vi "dcy06.vi"() -> ()   [LabVIEW 2015]
uses:
  SECoP.lvlib
  <vilib>/regexp/Match Regular Expression.xnode
  Public/SECoP-data/SECoP-data.ctl
  Public/SECoP-action.ctl
  parametertype.ctl
panel:
  out "log":string
  in  "DLL path":path=path "C:/Users/user/Desktop/x86_64"
  in  "stop":bool
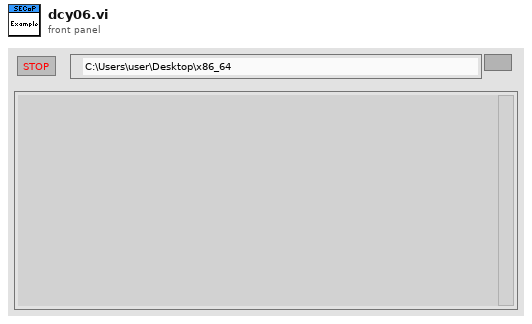
[diagram p1: front panel]
types:
  T1 = typedef "parametertype.ctl" = enum8{"readonly", "readwrite", "command"}
  T2 = typedef "SECoP.lvlib/SECoP-data.ctl" = cluster{"ptr32":u32, "ptr64":u64}
  T3 = cluster{"name":string, "type":T1, "datatype":string, "description":string, "SECoP_dataPtr":T2}[]
  T4 = typedef "SECoP.lvlib/SECoP-libraries.ctl" = cluster{"serverDLL":path, "variantDLL":path, "cleanup_mode":bool}
  T5 = cluster{"name":string, "type":T1, "datatype":string, "description":string, "SECoP_dataPtr":T2}
  T6 = typedef "SECoP.lvlib/SECoP-action.ctl" = enum32{"any action", "read", "change", "do cmd"}
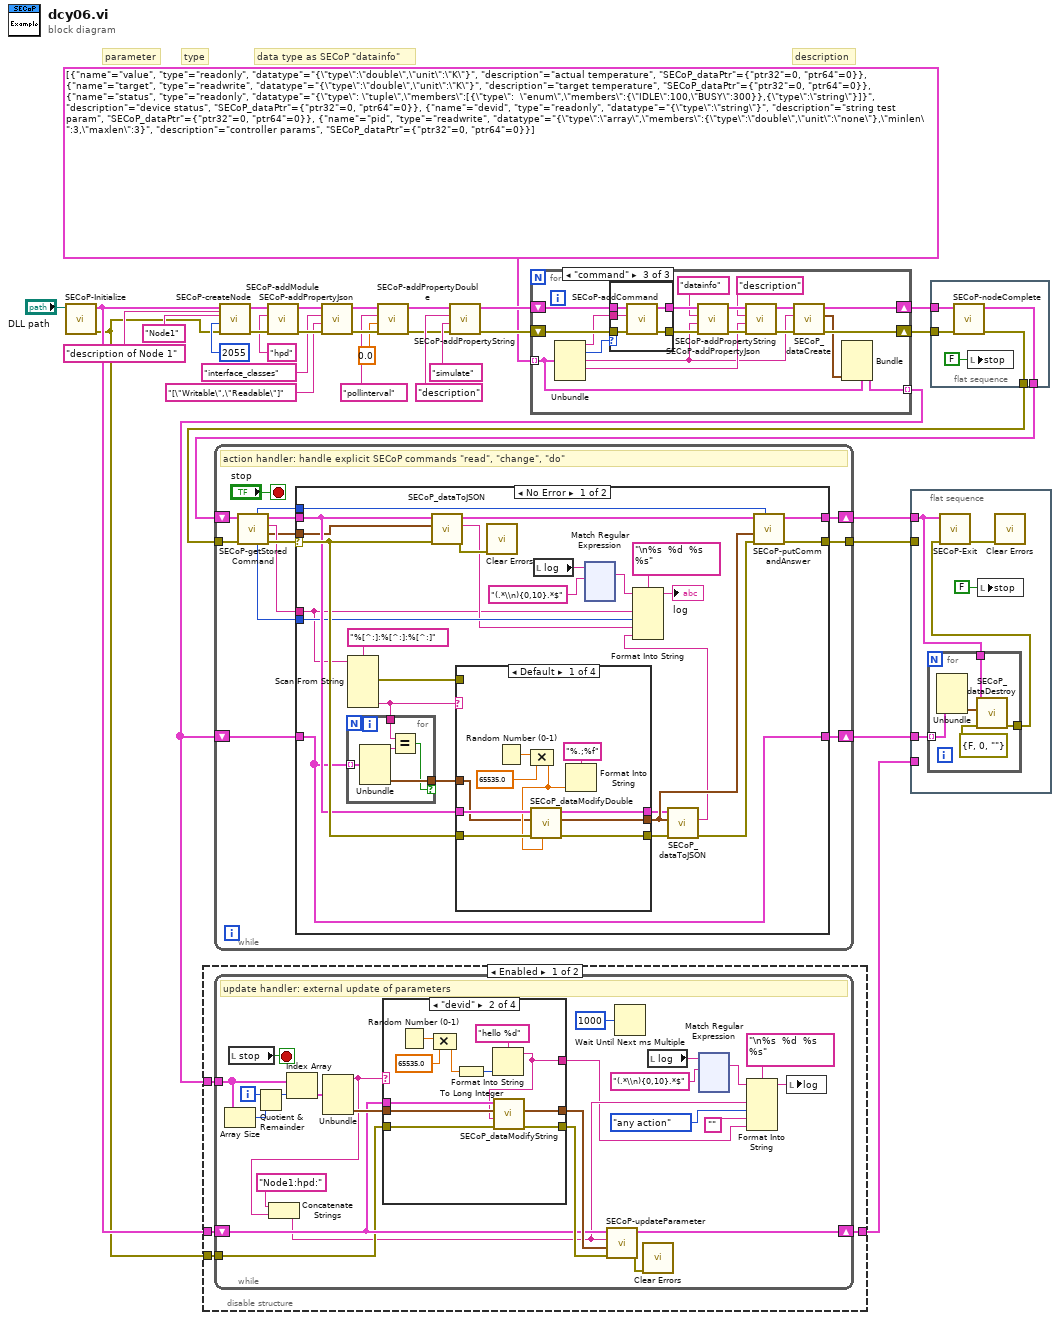
[diagram p0: block diagram]
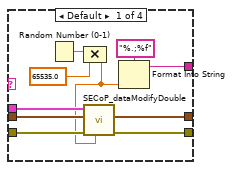
[diagram p2: hidden frame]
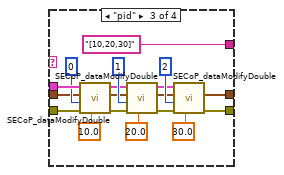
[diagram p3: hidden frame]
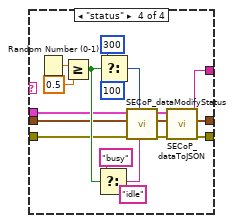
[diagram p4: hidden frame]
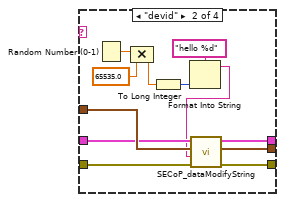
[diagram p6: hidden frame]
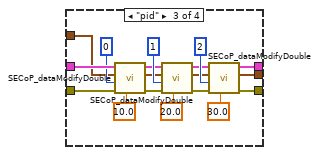
[diagram p7: hidden frame]
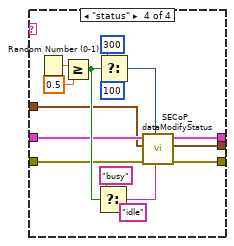
[diagram p8: hidden frame]
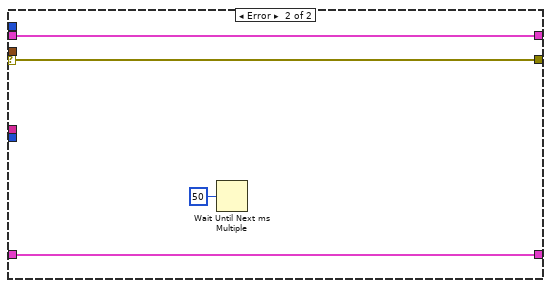
[diagram p9: hidden frame]
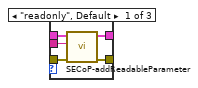
[diagram p10: hidden frame]
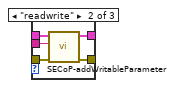
[diagram p11: hidden frame]
diagram:
  # "description"
  # "data type as SECoP \"datainfo\""
  # "type"
  # "parameter"
  n1 = call "SECoP-Initialize.vi"("DLL path (in)"="DLL path") -> ("error out"=w3:errorcluster, "DLL path (out)"=w4:T4)  [unwired: 9 in]
  n2 = call "SECoP-createNode.vi"("description"="description of Node 1", "error in (no error)"=w3, "TCP port"=u16 2055, "node id"="Node1" ("id"), "DLL path (in)"=w4) -> ("error out"=w28:errorcluster, "DLL path (out)"=w32:T4)  [unwired: 5 in]
  n3 = call "SECoP-addModule.vi"("error in (no error)"=w28, "module name"="hpd" ("name"), "DLL path (in)"=w32) -> ("error out"=w25:errorcluster, "DLL path (out)"=w26:T4)  [unwired: 7 in]
  n4 = call "SECoP-addPropertyJson.vi"("error in (no error)"=w25, "property value"="[\"Writable\",\"Readable\"]" ("name"), "property name"="interface_classes" ("name"), "DLL path (in)"=w26) -> ("error out"=w14:errorcluster, "DLL path (out)"=w16:T4)  [unwired: 6 in]
  n5 = call "SECoP-addPropertyDouble.vi"("error in (no error)"=w14, "property value"=0.0, "property name"="pollinterval", "DLL path (in)"=w16) -> ("error out"=w13:errorcluster, "DLL path (out)"=w15:T4)  [unwired: 6 in]
  n6 = call "SECoP-addPropertyString.vi"("error in (no error)"=w13, "property value"="simulate" ("name"), "property name"="description" ("name"), "DLL path (in)"=w15) -> ("error out"=w19:errorcluster, "DLL path (out)"=w20:T4)  [unwired: 6 in]
  n7 = for {
    tunnel: T3 [{"name"="value", "type"=enum."readonly", "datatype"="{\"type\":\"double\",\"unit\":\"K\"}", "description"="actual temperature", "SECoP_dataPtr"={"ptr32"=0, "ptr64"=0}}, {"name"="target", "type"=enum."readwrite", "datatype"="{\"type\":\"double\",\"unit\":\"K\"}", "description"="target temperature", "SECoP_dataPtr"={"ptr32"=0, "ptr64"=0}}, {"name"="status", "type"=enum."readonly", "datatype"="{\"type\": \"tuple\",\"members\":[{\"type\":  \"enum\",\"members\":{\"IDLE\":100,\"BUSY\":300}},{\"type\":\"string\"}]}", "description"="device status", "SECoP_dataPtr"={"ptr32"=0, "ptr64"=0}}, {"name"="devid", "type"=enum."readonly", "datatype"="{\"type\":\"string\"}", "description"="string test param", "SECoP_dataPtr"={"ptr32"=0, "ptr64"=0}}, {"name"="pid", "type"=enum."readwrite", "datatype"="{\"type\":\"array\",\"members\":{\"type\":\"double\",\"unit\":\"none\"},\"minlen\":3,\"maxlen\":3}", "description"="controller params", "SECoP_dataPtr"={"ptr32"=0, "ptr64"=0}}] -> [w36] mode=indexing
    shift-right: [w39] -> w8
    shift-left: w20 -> [w49]
    shift-right: [w38] -> w7
    shift-left: w19 -> [w48]
    tunnel: [w34] -> w1 mode=indexing
    n8 = Unbundle(w36) -> ("name"=w37:string, "type"=w50:T1, "datatype"=w40:string, "description"=w43:string)  [unwired: 1 out]
    n9 = case shown="\"command\"" w50 {
      tunnel: w37 -> [w55 w62 w67]
      tunnel: w49 -> [w57 w61 w66]
      tunnel: [w56 w60 w65] -> w47
      tunnel: [w53 w58 w63] -> w46
      tunnel: w48 -> [w54 w59 w64]
      frame "readonly", Default {
        n10 = call "SECoP-addReadableParameter.vi"("error in (no error)"=w54, "parameter name"=w55, "DLL path (in)"=w57) -> ("error out"=w53:errorcluster, "DLL path (out)"=w56:T4)  [unwired: 7 in]
      }
      frame "readwrite" {
        n11 = call "SECoP-addWritableParameter.vi"("error in (no error)"=w59, "parameter name"=w62, "DLL path (in)"=w61) -> ("error out"=w58:errorcluster, "DLL path (out)"=w60:T4)  [unwired: 7 in]
      }
      frame "command" {
        n12 = call "SECoP-addCommand.vi"("error in (no error)"=w64, "command name"=w67, "DLL path (in)"=w66) -> ("error out"=w63:errorcluster, "DLL path (out)"=w65:T4)  [unwired: 7 in]
      }
    }
    n13 = call "SECoP-addPropertyJson.vi"("error in (no error)"=w46, "property value"=w40, "property name"="datainfo" ("name"), "DLL path (in)"=w47) -> ("error out"=w51:errorcluster, "DLL path (out)"=w52:T4)  [unwired: 6 in]
    n14 = call "SECoP-addPropertyString.vi"("error in (no error)"=w51, "property value"=w43, "property name"="description" ("name"), "DLL path (in)"=w52) -> ("error out"=w42:errorcluster, "DLL path (out)"=w41:T4)  [unwired: 6 in]
    n15 = call "SECoP_dataCreate.vi"("error in (no error)"=w42, "Description"=w40, "DLL path (in)"=w41) -> ("error out"=w38:errorcluster, "SECoP_dataPtr (out)"=w35:T2, "DLL path (out)"=w39:T4)  [unwired: 6 in]
    n16 = Bundle(cluster=w36, "SECoP_dataPtr"=w35) -> (w34:T5)  [unwired: 4 in]
  }
  n17 = disable-structure shown="Enabled" {
    disable-tunnel: [w71 w261] -> w5
    disable-tunnel: w4 -> [w70 w261]
    disable-tunnel: w3 -> [w69 _]
    disable-tunnel: w1 -> [w68 _]
    frame Enabled {
      n18 = while {
        tunnel: w69 -> [w91]
        shift-right: [w90] -> w71
        shift-left: w70 -> [w92]
        tunnel: w68 -> [w81]
        i -> [w83]
        stop <- w93 stop-if-true
        # "update handler: external update of parameters"
        n19 = Array Size(array=w81) -> (size(s)=w84:i32)
        n20 = local read "stop"() -> (w93:bool)
        n21 = Quotient & Remainder(x=w83, y=w84) -> (x-y*floor(x/y)=w85:i32)  [unwired: 1 out]
        n22 = Index Array(array=w81, index=w85) -> (element=w82:T5)
        n23 = Unbundle(w82) -> ("name"=w88:string, "SECoP_dataPtr"=w94:T2)  [unwired: 3 out]
        n24 = Concatenate Strings("Node1:hpd:" ("string"), w88) -> (w76:string)
        n25 = case shown="\"devid\"" w88 {
          tunnel: [w215 w221 "[10,20,30]" w247] -> w74
          tunnel: w92 -> [w214 w225 w244 w252]
          tunnel: [w219 w222 w230 w250] -> w95
          tunnel: w91 -> [w213 w224 w242 w251]
          tunnel: [w212 w223 w231 w253] -> w96
          tunnel: w94 -> [w219 w222 w230 w250]
          frame Default {
            n26 = Random Number (0-1)() -> (number: 0 to 1=w217:dbl)
            n27 = Compound Arithmetic op=MULTIPLY(w217, 65535.0 ("value")) -> (w211:dbl)
            n28 = call "SECoP_dataModifyDouble.vi"("Value"=w211, "error in (no error)"=w213, "SECoP_data"=w219, "DLL path (in)"=w214) -> ("error out"=w212:errorcluster)  [unwired: 6 in, 1 out]
            n29 = Format Into String(format string="%.;%f", w211) -> (resulting string=w215:string)  [unwired: 2 in, 1 out]
          }
          frame "devid" {
            n30 = Random Number (0-1)() -> (number: 0 to 1=w226:dbl)
            n31 = Compound Arithmetic op=MULTIPLY(w226, 65535.0 ("value")) -> (w228:dbl)
            n32 = To Long Integer(number=w228) -> (32bit integer=w229:i32)
            n33 = Format Into String(format string="hello %d", w229) -> (resulting string=w221:string)  [unwired: 2 in, 1 out]
            n34 = call "SECoP_dataModifyString.vi"("error in (no error)"=w224, "Value"=w221, "SECoP_dataPtr"=w222, "DLL path (in)"=w225) -> ("error out"=w223:errorcluster)  [unwired: 6 in, 1 out]
          }
          frame "pid" {
            n35 = call "SECoP_dataModifyDouble.vi"("Value"=10.0, "error in (no error)"=w242, "Index"=u32 0, "SECoP_data"=w230, "DLL path (in)"=w244) -> ("error out"=w233:errorcluster, "DLL path (out)"=w235:T4)  [unwired: 5 in]
            n36 = call "SECoP_dataModifyDouble.vi"("Value"=20.0, "error in (no error)"=w233, "Index"=u32 1, "SECoP_data"=w230, "DLL path (in)"=w235) -> ("error out"=w232:errorcluster, "DLL path (out)"=w234:T4)  [unwired: 5 in]
            n37 = call "SECoP_dataModifyDouble.vi"("Value"=30.0, "error in (no error)"=w232, "Index"=u32 2, "SECoP_data"=w230, "DLL path (in)"=w234) -> ("error out"=w231:errorcluster)  [unwired: 5 in, 1 out]
          }
          frame "status" {
            n38 = Random Number (0-1)() -> (number: 0 to 1=w260:dbl)
            n39 = Greater Or Equal?(x=w260, y=0.5) -> (x >= y?=w256:bool)
            n40 = Select(t="busy", s=w256, f="idle") -> (s? t:f=w246:string)
            n41 = Select(t=i64 300 ("Value"), s=w256, f=i64 100 ("Value")) -> (s? t:f=w245:i64)
            n42 = call "SECoP_dataModifyStatus.vi"("status text"=w246, "status code"=w245, "error in (no error)"=w251, "SECoP_dataPtr (in)"=w250, "DLL path (in)"=w252) -> ("error out"=w248:errorcluster, "DLL path (out)"=w249:T4)  [unwired: 4 in, 1 out]
            n43 = call "SECoP_dataToJSON.vi"("error in (no error)"=w248, "SECoP_dataPtr"=w250, "DLL path (in)"=w249) -> ("error out"=w253:errorcluster, "JSONBuffer"=w247:string)  [unwired: 6 in, 1 out]
          }
        }
        n44 = call "SECoP-updateParameter.vi"("error in (no error)"=w96, "value (SECoP_data)"=w95, "parameter name"=w76, "DLL path (in)"=w92) -> ("error out"=w86:errorcluster, "DLL path (out)"=w90:T4)  [unwired: 6 in]
        n45 = Wait Until Next ms Multiple(millisecond multiple=u32 1000) -> ()  [unwired: 1 out]
        n46 = call <vilib>:"Clear Errors.vi"("error in (no error)"=w86) -> ()  [unwired: 5 in, 2 out]
        n47 = local read "log"() -> (w80:string)
        n48 = xnode "Match Regular Expression"("input string"=w80, "regular expression"="(.*\\n){0,10}.*$") -> ("whole match"=w79:string)  [unwired: 4 in, 4 out]
        n49 = Format Into String(format string="\n%s  %d  %s  %s", initial string=w79, w76, SECoP-action."any action" ("input 2"), "", w74) -> (resulting string=w72:string)  [unwired: 1 in, 1 out]
        n50 = local write "log"(w72) -> ()
      }
    }
    frame Disabled {
    }
  }
  n51 = while {
    shift-right: [w274] -> w22
    shift-left: w9 -> [w272]
    tunnel: w10 -> [w271]
    tunnel: [w264] -> w21
    shift-right: [w262] -> w6
    shift-left: w1 -> [w263]
    stop <- "stop" stop-if-true
    # "action handler: handle explicit SECoP commands \"read\", \"change\", \"do\""
    n52 = call "SECoP-getStoredCommand.vi"("error in (no error)"=w271, "DLL path (in)"=w272) -> ("error out"=w269:errorcluster, "SECoP_data"=w265:T2, "command/parameter path"=w266:string, "DLL path (out)"=w270:T4, "action"=w267:T6, "command id"=w268:u64)  [unwired: 4 in]
    n53 = case shown="No Error" w269 {
      selector: w269 -> [w299 w471]
      tunnel: w270 -> [w298 w472]
      tunnel: [w295 w472] -> w274
      tunnel: w268 -> [w294 _]
      tunnel: w266 -> [w283 _]
      tunnel: w265 -> [w280 _]
      tunnel: w267 -> [w293 _]
      tunnel: [w296 w471] -> w264
      tunnel: w263 -> [w279 w470]
      tunnel: [w279 w470] -> w262
      frame No Error {
        n54 = Scan From String(format string="%[^:]:%[^:]:%[^:]", input string=w283) -> (error out=w287:errorcluster, output 3=w282:string)  [unwired: 7 in, 2 out]
        n55 = for {
          tunnel: w279 -> [w301] mode=indexing
          tunnel: w282 -> [w304]
          tunnel: [w303] -> w281 if=w302
          n56 = Unbundle(w301) -> ("name"=w305:string, "SECoP_dataPtr"=w303:T2)  [unwired: 3 out]
          n57 = Equal?(x=w304, y=w305) -> (x = y?=w302:bool)
        }
        n58 = call "SECoP_dataToJSON.vi"("error in (no error)"=w299, "SECoP_dataPtr"=w280, "DLL path (in)"=w298) -> ("error out"=w297:errorcluster, "JSONBuffer"=w284:string, "DLL path (out)"=w285:T4)  [unwired: 6 in]
        n59 = case shown="Default" w282 {
          tunnel: w287 -> [_ _ _ _]
          tunnel: w298 -> [w311 w319 w340 w347]
          tunnel: [w307 w325 w327 w345] -> w300
          tunnel: w299 -> [w310 w318 w339 w346]
          tunnel: [w309 w316 w328 w342] -> w276
          tunnel: w281 -> [w307 w325 w327 w345]
          tunnel: [w306 w315 w326 w341] -> w277
          frame Default {
            n60 = Random Number (0-1)() -> (number: 0 to 1=w313:dbl)
            n61 = Compound Arithmetic op=MULTIPLY(w313, 65535.0 ("value")) -> (w308:dbl)
            n62 = call "SECoP_dataModifyDouble.vi"("Value"=w308, "error in (no error)"=w310, "SECoP_data"=w307, "DLL path (in)"=w311) -> ("error out"=w309:errorcluster, "DLL path (out)"=w306:T4)  [unwired: 6 in]
            n63 = Format Into String(format string="%.;%f", w308) -> ()  [unwired: 2 in, 2 out]
          }
          frame "devid" {
            n64 = Random Number (0-1)() -> (number: 0 to 1=w321:dbl)
            n65 = Compound Arithmetic op=MULTIPLY(w321, 65535.0 ("value")) -> (w323:dbl)
            n66 = To Long Integer(number=w323) -> (32bit integer=w324:i32)
            n67 = Format Into String(format string="hello %d", w324) -> (resulting string=w317:string)  [unwired: 2 in, 1 out]
            n68 = call "SECoP_dataModifyString.vi"("error in (no error)"=w318, "Value"=w317, "SECoP_dataPtr"=w325, "DLL path (in)"=w319) -> ("error out"=w316:errorcluster, "DLL path (out)"=w315:T4)  [unwired: 6 in]
          }
          frame "pid" {
            n69 = call "SECoP_dataModifyDouble.vi"("Value"=10.0, "error in (no error)"=w339, "Index"=u32 0, "SECoP_data"=w327, "DLL path (in)"=w340) -> ("error out"=w330:errorcluster, "DLL path (out)"=w332:T4)  [unwired: 5 in]
            n70 = call "SECoP_dataModifyDouble.vi"("Value"=20.0, "error in (no error)"=w330, "Index"=u32 1, "SECoP_data"=w327, "DLL path (in)"=w332) -> ("error out"=w329:errorcluster, "DLL path (out)"=w331:T4)  [unwired: 5 in]
            n71 = call "SECoP_dataModifyDouble.vi"("Value"=30.0, "error in (no error)"=w329, "Index"=u32 2, "SECoP_data"=w327, "DLL path (in)"=w331) -> ("error out"=w328:errorcluster, "DLL path (out)"=w326:T4)  [unwired: 5 in]
          }
          frame "status" {
            n72 = Random Number (0-1)() -> (number: 0 to 1=w354:dbl)
            n73 = Greater Or Equal?(x=w354, y=0.5) -> (x >= y?=w350:bool)
            n74 = Select(t="busy", s=w350, f="idle") -> (s? t:f=w344:string)
            n75 = Select(t=i64 300 ("Value"), s=w350, f=i64 100 ("Value")) -> (s? t:f=w343:i64)
            n76 = call "SECoP_dataModifyStatus.vi"("status text"=w344, "status code"=w343, "error in (no error)"=w346, "SECoP_dataPtr (in)"=w345, "DLL path (in)"=w347) -> ("error out"=w342:errorcluster, "DLL path (out)"=w341:T4)  [unwired: 4 in, 1 out]
          }
        }
        n77 = call <vilib>:"Clear Errors.vi"("error in (no error)"=w297) -> ()  [unwired: 5 in, 2 out]
        n78 = local read "log"() -> (w290:string)
        n79 = xnode "Match Regular Expression"("input string"=w290, "regular expression"="(.*\\n){0,10}.*$") -> ("whole match"=w291:string)  [unwired: 4 in, 4 out]
        n80 = call "SECoP_dataToJSON.vi"("error in (no error)"=w276, "SECoP_dataPtr"=w300, "DLL path (in)"=w277) -> ("error out"=w275:errorcluster, "JSONBuffer"=w278:string)  [unwired: 6 in, 1 out]
        n81 = Format Into String(format string="\n%s  %d  %s  %s", initial string=w291, w283, w293, w284, w278) -> (resulting string=→"log":string)  [unwired: 1 in, 1 out]
        n82 = call "SECoP-putCommandAnswer.vi"("command id"=w294, "error in (no error)"=w275, "value (SECoP_data)"=w300, "DLL path (in)"=w285) -> ("error out"=w296:errorcluster, "DLL path (out)"=w295:T4)  [unwired: 6 in]
      }
      frame Error {
        n83 = Wait Until Next ms Multiple(millisecond multiple=u32 50) -> ()  [unwired: 1 out]
      }
    }
  }
  n84 = flat-sequence {
    tunnel: w22 -> [w474]
    tunnel: w21 -> [_]
    tunnel: w6 -> [w476]
    tunnel: w5 -> [_]
    frame #0 {
      n85 = for {
        tunnel: w476 -> [w482] mode=indexing
        tunnel: [w480] -> w475
        tunnel: w474 -> [w479]
        n86 = Unbundle(w482) -> ("SECoP_dataPtr"=w481:T2)  [unwired: 4 out]
        n87 = call "SECoP_dataDestroy.vi"("error in (no error)"=errorcluster {"status"=FALSE, "code"=0, "source"=""}, "SECoP_dataPtr"=w481, "DLL path (in)"=w479) -> ("error out"=w480:errorcluster)  [unwired: 7 in, 1 out]
      }
      n88 = call "SECoP-Exit.vi"("error in (no error)"=w475, "DLL path (in)"=w474) -> ("error out"=w473:errorcluster)  [unwired: 9 in]
      n89 = local write "stop"(FALSE) -> ()
      n90 = call <vilib>:"Clear Errors.vi"("error in (no error)"=w473) -> ()  [unwired: 5 in, 2 out]
    }
  }
  n91 = flat-sequence {
    tunnel: w8 -> [w486]
    tunnel: w7 -> [w485]
    tunnel: [w483] -> w9
    tunnel: [w484] -> w10
    frame #0 {
      n92 = call "SECoP-nodeComplete.vi"("error in (no error)"=w485, "DLL path (in)"=w486) -> ("error out"=w484:errorcluster, "DLL path (out)"=w483:T4)  [unwired: 8 in]
      n93 = local write "stop"(FALSE) -> ()
    }
  }
